vi "globale bedingungen.vi"   [LabVIEW 2010]
uses:
  pertrasgc fpga/gvbooleschRT.vi
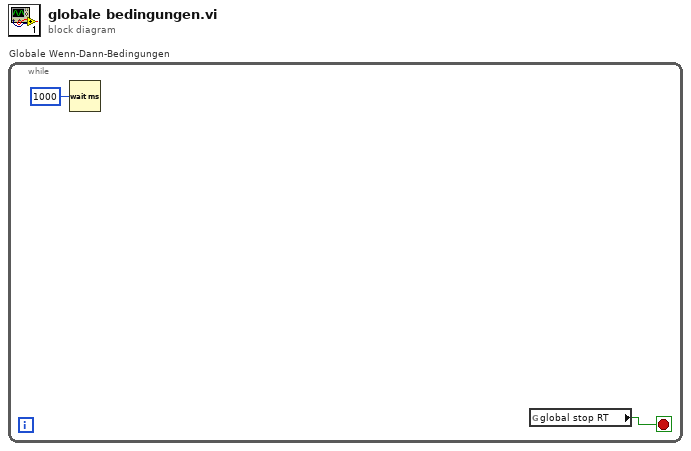
[diagram p0: block diagram]
diagram:
  n1 = while "Globale Wenn-Dann-Bedingungen" {
    stop <- w2 stop-if-true
    n2 = Wait (ms)(milliseconds to wait=u32 1000 ("Zu wartende ms")) -> ()  [unwired: 1 out]
    n3 = global read "gvbooleschRT.vi" "global stop RT"() -> (w2:bool)
  }
